vi "Set Debug Options.vi"(8 "error in":errorcluster, 9 "infinite FIFO timeouts":bool, 10 "debug":bool, 11 "data sharing framework custom device in":T1 format="%.0x") -> (0 "error out":errorcluster, 3 "data sharing framework custom device out":T1 format="%.0x")   [LabVIEW 2020, in "Data Sharing Framework Custom Device Scripting.lvlib"]
doc: "Writes the <b>debug</b> and <b>infinite FIFO timeouts</b> options. These options are available for all targets."
uses:
  Data Sharing Framework Custom Device Scripting.lvlib
  <vilib>/NI VeriStand/Custom Device API/Custom Device Item Ref.ctl
  DSF Shared.lvlib
  <vilib>/NI VeriStand/Custom Device API/Custom Device API.lvlib
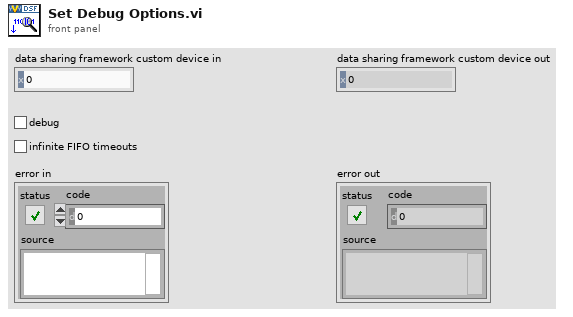
[diagram p1: front panel]
types:
  T1 = typedef "Custom Device API.lvlib/Custom Device Item Ref.ctl" = u64
  T2 = typedef "DSF Core.lvlibp/Framework.lvclass/Framework Options.ctl" = cluster{"FIFO Options":T3, "Thread Options":T4, "Plugin Options":T5, "Performance Options":T6, "Data Server Options":T7}
  T3 = typedef "DSF Core.lvlibp/Framework.lvclass/DSF FIFO Options.ctl" = cluster{"Infinite Timeouts":bool}
  T4 = typedef "DSF Core.lvlibp/Thread.lvclass/Thread Options.ctl" = cluster{"Show FP On Call":bool, "Close FP After Call":bool, "Allow Debugging":bool}
  T5 = typedef "DSF Core.lvlibp/Framework.lvclass/DSF Plugin Options.ctl" = cluster{"Default Components":bool}
  T6 = typedef "DSF Core.lvlibp/DSF Performance Options.ctl" = cluster{"Measure Period":bool, "Measure Rx/Tx Duration":bool}
  T7 = typedef "DSF Core.lvlibp/Framework.lvclass/Data Server Options.ctl" = cluster{"Enable Data Server":bool, "Period":u32}
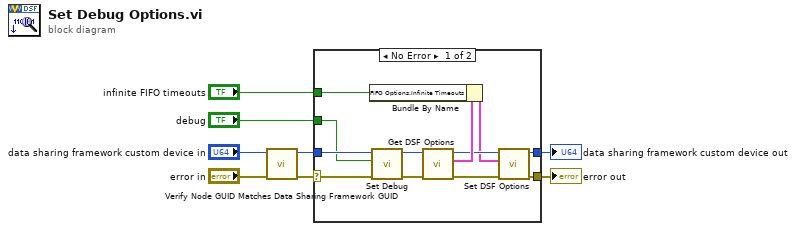
[diagram p0: block diagram]
diagram:
  n1 = call "Verify Node GUID Matches Data Sharing Framework GUID.vi"("error in"="error in", "data sharing framework custom device in"="data sharing framework custom device in") -> ("error out"=w1:errorcluster, "data sharing framework custom device out"=w2:T1)  [unwired: 8 in]
  n2 = case shown="No Error" w1 {
    selector: w1 -> [w13 w21]
    tunnel: "debug" -> [w9 _]
    tunnel: "infinite FIFO timeouts" -> [w19 _]
    tunnel: [w16 w22] -> w6
    tunnel: [w15 w21] -> w5
    tunnel: w2 -> [w10 w22]
    frame No Error {
      n3 = call "Set Debug.vi"("error in (no error)"=w13, "debug"=w9, "Item Ref in"=w10) -> ("error out"=w12:errorcluster, "Item Ref out"=w11:T1)  [unwired: 7 in]
      n4 = call "Get DSF Options.vi"("error in (no error)"=w12, "Item Ref in"=w11) -> ("error out"=w17:errorcluster, "options"=w20:T2, "Item Ref out"=w18:T1)  [unwired: 7 in]
      n5 = Bundle By Name(cluster=w20, "FIFO Options.Infinite Timeouts"=w19) -> (w14:T2)
      n6 = call "Set DSF Options.vi"("error in (no error)"=w17, "options"=w14, "Item Ref in"=w18) -> ("error out"=w15:errorcluster, "Item Ref out"=w16:T1)  [unwired: 7 in]
    }
    frame Error {
    }
  }
  "data sharing framework custom device out" <- w6
  "error out" <- w5
